vi "DriveDistance.vi"(8 "Start Drive Straight (Hold)":bool=TRUE, 9 "Negate":bool, 10 "Drive PID":T1={"proportional gain (Kc)"=1.0, "integral time (Ti, min)"=0.01, "derivative time (Td, min)"=0.0} {"derivative time (Td, min)" format="%.3f"; "integral time (Ti, min)" format="%.3f"; "proportional gain (Kc)" format="%.3f"}, 11 "Drive Values":T2 {"Throttle Scale" scale=0.0..1.0}) -> (1 "Distance Remaining":dbl, 3 "Cheesy Throttle":dbl)   [LabVIEW 2015]
uses:
  <vilib>/addons/control/pid/pid.llb/PID (DBL).vi
  <vilib>/addons/control/pid/NI_PID_pid.lvlib
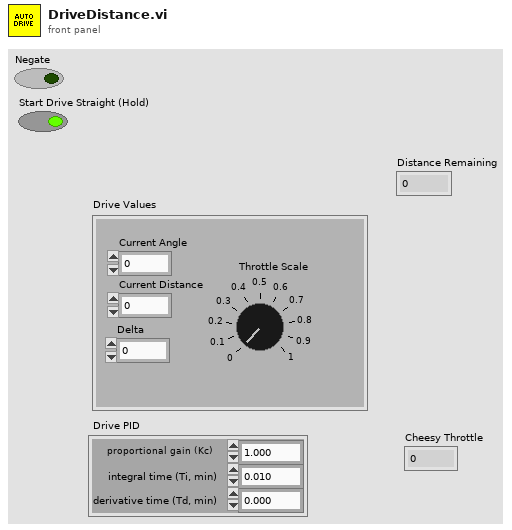
[diagram p1: front panel]
types:
  T1 = cluster{"proportional gain (Kc)":dbl, "integral time (Ti, min)":dbl, "derivative time (Td, min)":dbl}
  T2 = cluster{"Delta":dbl, "Throttle Scale":dbl, "Current Angle":dbl, "Current Distance":dbl}
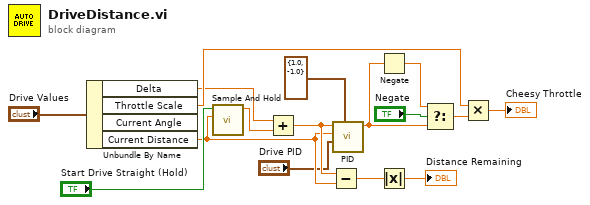
[diagram p0: block diagram]
diagram:
  n1 = Unbundle By Name("Drive Values") -> ("Delta"=w3:dbl, "Throttle Scale"=w8:dbl, "Current Distance"=w6:dbl)  [unwired: 1 out]
  n2 = call "Sample And Hold.vi"("Signal"=w6, "Condition"="Start Drive Straight (Hold)") -> ("Signal Out"=w15:dbl)  [unwired: 9 in]
  n3 = Add(x=w3, y=w15) -> (x+y=w7:dbl)
  n4 = Subtract(x=w7, y=w6) -> (x-y=w5:dbl)
  n5 = call-poly <vilib>:"PID.vi"("output range"=cluster{"output high":dbl, "output low":dbl} {"output high"=1.0, "output low"=-1.0}, "PID gains"="Drive PID", "process variable"=w6, "setpoint"=w7) -> ("output"=w13:dbl)  [unwired: 6 in, 1 out]
  n6 = Negate(x=w13) -> (-x=w14:dbl)
  n7 = Absolute Value(x=w5) -> (abs(x)=→"Distance Remaining":dbl)
  n8 = Select(t=w14, s="Negate", f=w13) -> (s? t:f=w11:dbl)
  n9 = Multiply(x=w8, y=w11) -> (x*y=→"Cheesy Throttle":dbl)
